vi "Run VBAI.vi"(8 "error in":errorcluster, 9 "SN":string, 10 "Path":string="C:\\Tmp", 11 "VBAI":cluster{"New Image":T1, "VBAI Session Out":T2}) -> (0 "error out":errorcluster, 2 "Result":bool, 3 "Defect identify data":cluster{"Image":T1, "Measure Report":string})   [LabVIEW 2018]
uses:
  <vilib>/vision/Image Controls.llb/IMAQ Image.ctl
  <vilib>/userdefined/High Color/VBAIInterface.ctl
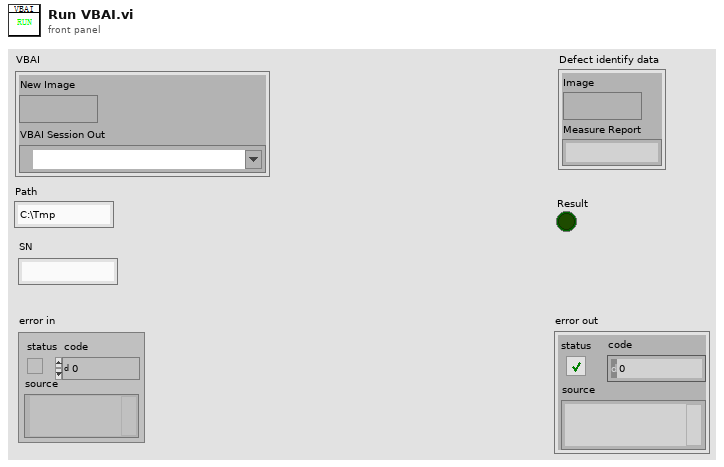
[diagram p1: front panel]
types:
  T1 = typedef "IMAQ Image.ctl" = refnum<image>
  T2 = typedef "VBAIInterface.ctl" = refnum<k21>
  T3 = enum16{"No Saved", "All Saved", "Only Fail Saved"}
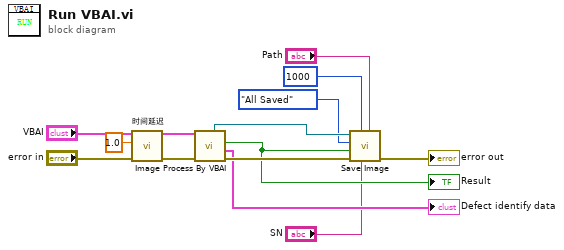
[diagram p0: block diagram]
diagram:
  n1 = call "时间延迟"("error in (no error)"="error in", "Delay Time (s)"=1.0) -> ("error out"=w5:errorcluster)  [unwired: 9 in]
  n2 = call "Image Process By VBAI.vi"("error in"=w5, "VBAI"="VBAI") -> ("error out"=w13:errorcluster, "Defect identify data"=→"Defect identify data":cluster{"Image":T1, "Measure Report":string}, "Result"=w9:bool, "Image"=w12:T1)  [unwired: 4 in, 2 out]
  "Result" <- w9
  n3 = call "Save Image.vi"("Path"="Path", "SN"="SN", "Image Quality"=u32 1000, "error in (no error)"=w13, "PassFail"=w9, "Image Saved"=T3."All Saved", "Image"=w12) -> ("error out"=→"error out":errorcluster)  [unwired: 4 in]
